vi "Controller Write BPM or PS Filter Enable.vi"(0 "BPM-PS Filter Enable":refnum<k21>[](array[refnum]), 5 "Filter Enable":bool, 11 "error in":errorcluster) -> (15 "error out":errorcluster)   [LabVIEW 2011, in "Controller VIs.lvlib"]
uses:
  Controller VIs.lvlib
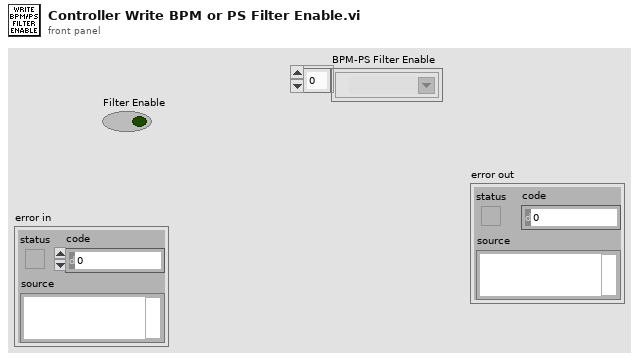
[diagram p1: front panel]
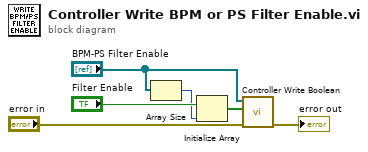
[diagram p0: block diagram]
diagram:
  n1 = Array Size(array="BPM-PS Filter Enable") -> (size(s)=w2:i32)
  n2 = Initialize Array("Filter Enable", w2) -> (w3:bool[])
  n3 = call "Controller Write Boolean.vi"("Error In"="error in", "Values"=w3, "Variables"="BPM-PS Filter Enable") -> ("Error Out"=→"error out":errorcluster)  [unwired: 8 in]
